vi "Start Create.vi"(9 "Alias":string, 10 "Actor":refnum<class "Actor.lvclass">, 11 "Base Actor in":refnum<class "Base Actor.lvclass">) -> (0 "Error out":errorcluster, 3 "Base Actor out":refnum<class "Base Actor.lvclass">)   [LabVIEW 2020, in "jettl.lvlib" / "Actor.lvlib" / "Base Actor.lvclass"]
uses:
  Base Actor.lvclass
  Actor/Actor.lvclass
  Attributes/Attributes/Attributes.lvclass
  Base Actor.lvclass/Base Actor.ctl
  Actor.lvlib
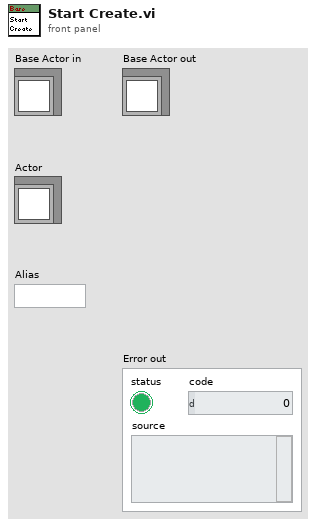
[diagram p1: front panel]
types:
  T1 = typedef "jettl.lvlib/Actor.lvlib/Base Actor.lvclass/Created Attributes Map.ctl" = map{string, refnum<class "Attributes.lvclass">}
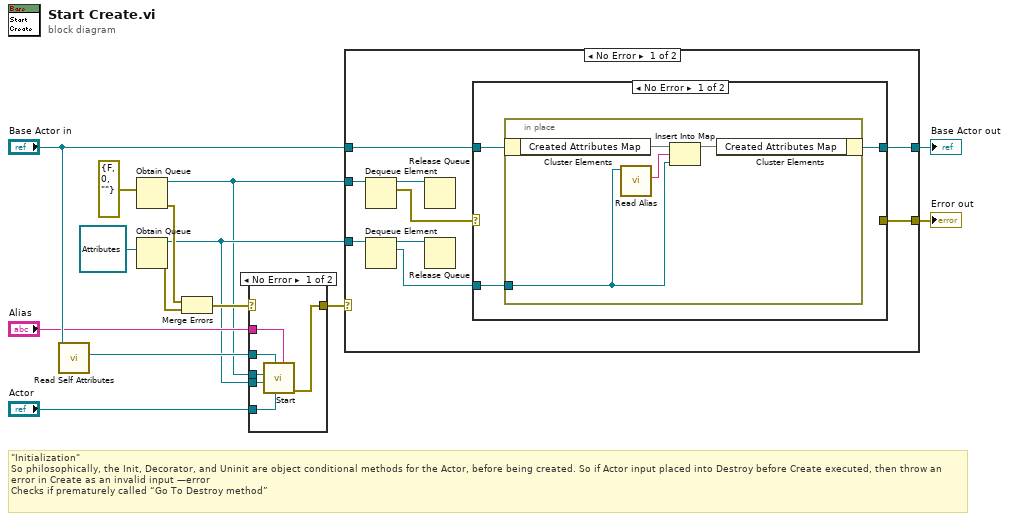
[diagram p0: block diagram]
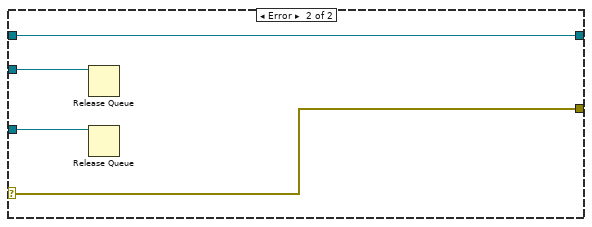
[diagram p4: hidden frame]
diagram:
  # "\"Initialization\"\nSo philosophically, the Init, Decorator, and Uninit are object conditional methods for the Actor, before being created. So if Actor input placed into Destroy before Create executed, then throw an error in Create as an invalid input —error  \nChecks if prematurely called “Go To Destroy method”"
  n1 = call-dynamic "Read Self Attributes.vi"("Base Actor in"="Base Actor in") -> ("Self Attributes"=w7:refnum<class "Attributes.lvclass">)  [unwired: 10 in]
  n2 = Obtain Queue(element data type=errorcluster {"status"=FALSE, "code"=0, "source"=""} ("Error")) -> (queue out=w1:refnum<queue>, error out=w3:errorcluster)  [unwired: 4 in, 1 out]
  n3 = Obtain Queue(element data type=refnum<class "Attributes.lvclass"> refnum ("jettl.lvlib:Attributes.lvlib:Attributes.lvclass")) -> (queue out=w2:refnum<queue>, error out=w9:errorcluster)  [unwired: 4 in, 1 out]
  n4 = Merge Errors(w3, w9) -> (w4:errorcluster)
  n5 = case shown="No Error" w4 {
    selector: w4 -> [_ w21]
    tunnel: "Alias" -> [w17 _]
    tunnel: w7 -> [w16 _]
    tunnel: w2 -> [w19 _]
    tunnel: [w20 w21] -> w8
    tunnel: w1 -> [w18 _]
    tunnel: "Actor" -> [w15 _]
    frame No Error {
      n6 = call "Start.vi"("Alias"=w17, "Actor"=w15, "Creator Attributes"=w16, "Queue of Self Attributes"=w19, "Queue of Error"=w18) -> ("Error out"=w20:errorcluster)  [unwired: 6 in]
    }
    frame Error {
    }
  }
  n7 = case shown="No Error" w8 {
    selector: w8 -> [_ w40]
    tunnel: "Base Actor in" -> [w30 w42]
    tunnel: [w29 w42] -> w14
    tunnel: w2 -> [w28 w43]
    tunnel: w1 -> [w26 w41]
    tunnel: [w22 w40] -> w12
    frame No Error {
      n8 = Dequeue Element(queue=w26) -> (queue out=w25:refnum<queue>, element=w23:errorcluster)  [unwired: 2 in, 2 out]
      n9 = Dequeue Element(queue=w28) -> (queue out=w27:refnum<queue>, element=w24:refnum<class "Attributes.lvclass">)  [unwired: 2 in, 2 out]
      n10 = Release Queue(queue=w25) -> ()  [unwired: 2 in, 3 out]
      n11 = Release Queue(queue=w27) -> ()  [unwired: 2 in, 3 out]
      n12 = case shown="No Error" w23 {
        selector: w23 -> [_ w38]
        tunnel: w30 -> [w32 w39]
        tunnel: [w31 w39] -> w29
        tunnel: w24 -> [w33 _]
        tunnel: [_ w38] -> w22
        frame No Error {
          n13 = in-place {
            in-place-border: w33 -> [w34]
            n14 = in-place-cluster #1(w32) -> ("Created Attributes Map"=w37:T1)
            n15 = call-dynamic "Read Alias.vi"("Attributes in"=w34) -> ("Alias"=w35:string)  [unwired: 10 in]
            n16 = Insert Into Map(map in=w37, key=w35, value=w34) -> (map out=w36:T1)  [unwired: 2 out]
            n17 = in-place-cluster #1("Created Attributes Map"=w36) -> (w31:refnum<class "Base Actor.lvclass">)
          }
        }
        frame Error {
        }
      }
    }
    frame Error {
      n18 = Release Queue(queue=w41) -> ()  [unwired: 2 in, 3 out]
      n19 = Release Queue(queue=w43) -> ()  [unwired: 2 in, 3 out]
    }
  }
  "Base Actor out" <- w14
  "Error out" <- w12
